vi "Cleanup Session.vi"(8 "error in":errorcluster, 11 "Plugin in":refnum<class "Tone Measurements.lvclass">) -> (0 "error out":errorcluster, 3 "Plugin out":refnum<class "Tone Measurements.lvclass">)   [LabVIEW 2025, in "Tone Measurements.lvlib" / "Tone Measurements.lvclass"]
uses:
  Tone Measurements.lvclass
  Tone Measurements.lvclass/Tone Measurements.ctl
  <vilib>/addons/_NISVFA/_Shared subVIs/Data Objects/Waveforms (DBL)/Waveforms (N Ch).lvclass
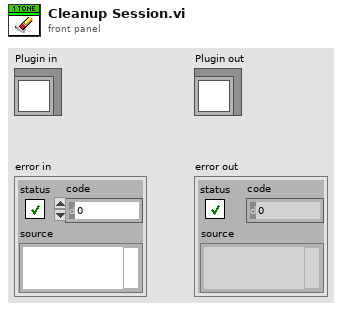
[diagram p1: front panel]
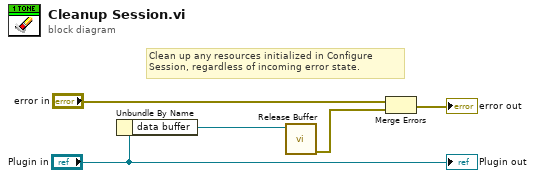
[diagram p0: block diagram]
diagram:
  # "Clean up any resources initialized in Configure Session, regardless of incoming error state."
  n1 = Unbundle By Name("Plugin in") -> ("data buffer"=w2:refnum<data-value>)
  n2 = call <vilib>:"Release Buffer.vi"("buffer"=w2) -> ("error out"=w1:errorcluster)  [unwired: 10 in]
  n3 = Merge Errors("error in", w1) -> (→"error out":errorcluster)
  "Plugin out" <- "Plugin in"
